vi "ScanAction.vi"(8 "error in (no error)":errorcluster caption="entrée d'erreur (pas d'erreur)", 9 "IndicePoint":i32, 11 "Dev In":refnum<class "KlingerMotor.lvclass"> caption="DNL_LabVIEW Object in") -> (0 "error out":errorcluster caption="sortie d'erreur", 2 "ScanParsOut":dbl[](array[numeric]), 3 "Dev Out":refnum<class "KlingerMotor.lvclass"> caption="DNL_LabVIEW Object out")   [LabVIEW 2012, in "KlingerMotor.lvclass"]
uses:
  KlingerMotor.lvclass
  KlingerMotor.lvclass/KlingerMotor.ctl
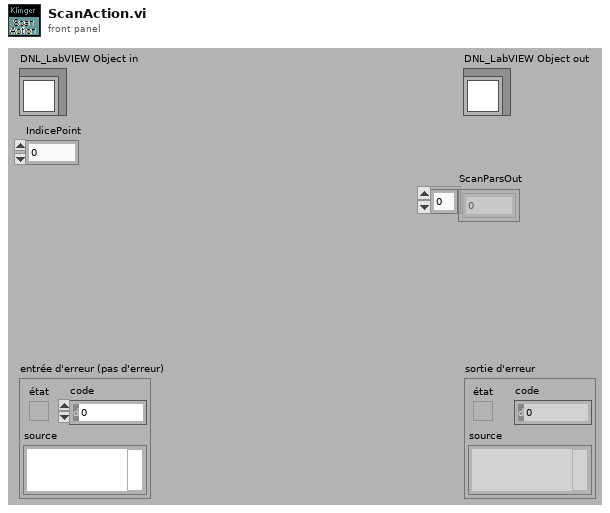
[diagram p1: front panel]
types:
  T1 = cluster{"Position Ref":refnum<vi>, "Moving Ref":refnum<vi>, "PLimRef":refnum<vi>, "NLimRef":refnum<vi>}
  T2 = typedef "KlingerMotor.lvclass/KlingerMotor_Func.ctl" = enum16{"Positions (mm)", "Position (ps)", "ReadWPos (ps)", "ReadWPos (mm)", "ReadZPos (ps)", "ReadZPos (mm)"}
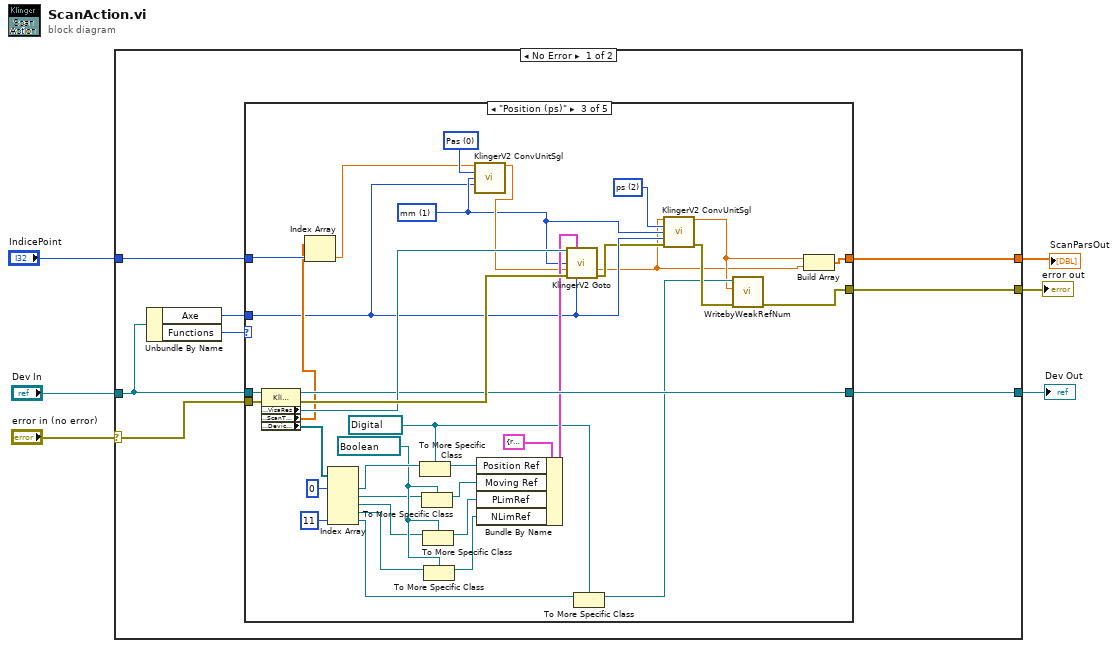
[diagram p0: block diagram]
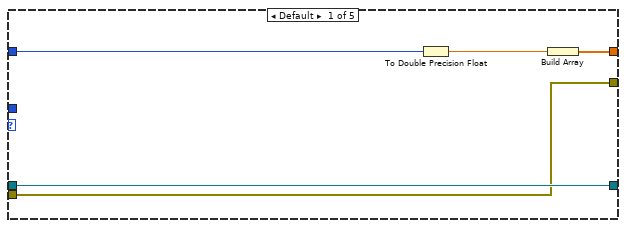
[diagram p2: hidden frame]
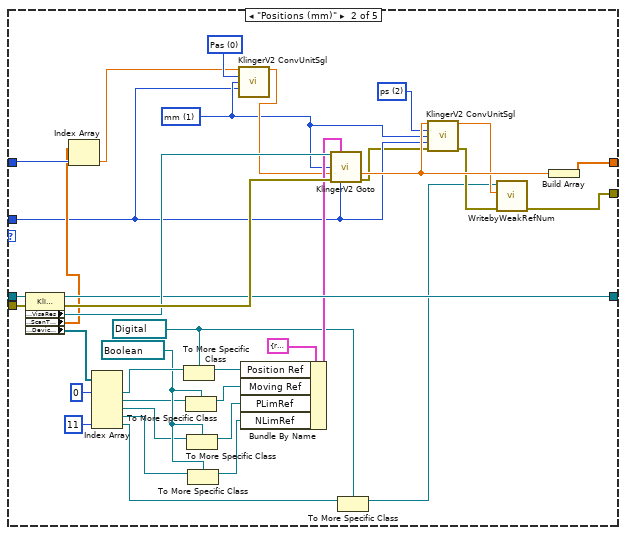
[diagram p3: hidden frame]
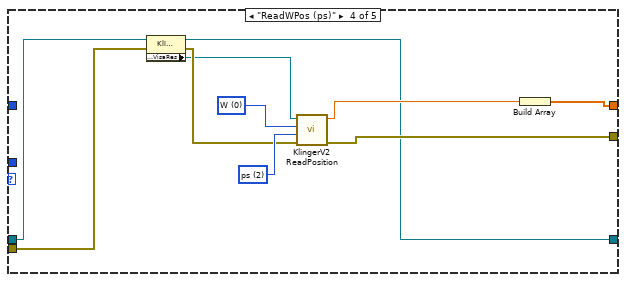
[diagram p4: hidden frame]
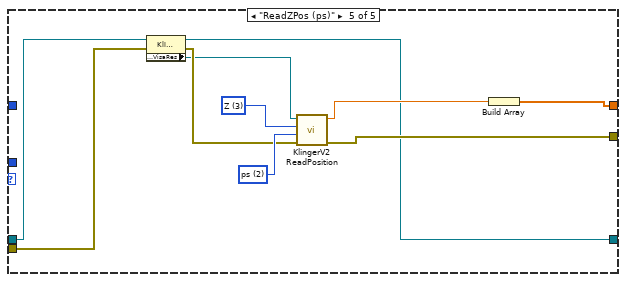
[diagram p5: hidden frame]
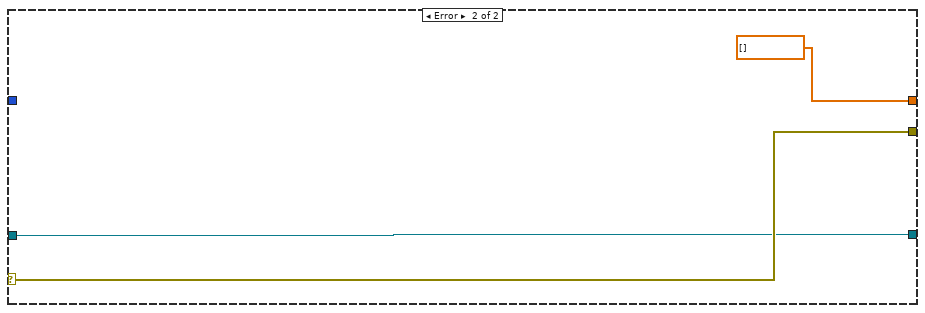
[diagram p6: hidden frame]
diagram:
  n1 = case shown="No Error" "error in (no error)" {
    selector: "error in (no error)" -> [w11 w114]
    tunnel: "Dev In" -> [w12 w113]
    tunnel: [w10 dbl[] []] -> w1
    tunnel: [w9 w114] -> w4
    tunnel: [w8 w113] -> w3
    tunnel: "IndicePoint" -> [w13 _]
    frame No Error {
      n2 = Unbundle By Name(w12) -> ("Axe"=w7:u8, "Functions"=w14:T2)
      n3 = case shown="\"Position (ps)\"" w14 {
        tunnel: [w15 w20 w57 w92 w102] -> w10
        tunnel: w13 -> [w19 w51 w87 _ _]
        tunnel: [w17 w50 w86 w93 w103] -> w8
        tunnel: w12 -> [w17 w55 w91 w96 w106]
        tunnel: w11 -> [w16 w54 w90 w97 w107]
        tunnel: [w16 w25 w62 w94 w104] -> w9
        tunnel: w7 -> [_ w29 w66 _ _]
        frame Default {
          n4 = To Double Precision Float(number=w19) -> (double precision float=w18:dbl)
          n5 = Build Array(w18) -> (w15:dbl[])
        }
        frame "Positions (mm)" {
          w31 = u8 2 items=["Pas", "mm", "ps", "Degré (°)"] ("UnitDem")
          w35 = u8 0 items=["Pas", "mm", "ps", "Degré (°)"] ("UnitDem")
          w42 = refnum<vi> refnum ("Moving Ref")
          w22 = refnum<vi> refnum ("Position Ref")
          w30 = u8 1 items=["Pas", "mm", "ps"] ("UnitDem")
          n6 = property class="KlingerMotor.lvclass"(reference=w55, error in=w54) -> (reference out=w50:refnum<class "KlingerMotor.lvclass">, error out=w53:errorcluster, "Accessor:VisaRes"=w52:refnum<visa-resource-name>, "Accessor:ScanTable"=w49:dbl[], "Accessor:DeviceCtrl"=w46:refnum<vi>[])
          n7 = Index Array(array=w49, index=w51) -> (element=w34:dbl)
          n8 = Index Array(array=w46, index #1=0 ("index"), index #5=11 ("index")) -> (element #1=w45:refnum<vi>, element #2=w41:refnum<vi>, element #3=w40:refnum<vi>, element #4=w39:refnum<vi>, element #5=w23:refnum<vi>)  [unwired: 3 in]
          n9 = To More Specific Class(target class=w22, reference=w45) -> (specific class reference=w43:refnum<vi>)  [unwired: 1 in, 1 out]
          n10 = To More Specific Class(target class=w42, reference=w41) -> (specific class reference=w38:refnum<vi>)  [unwired: 1 in, 1 out]
          n11 = To More Specific Class(target class=w42, reference=w40) -> (specific class reference=w37:refnum<vi>)  [unwired: 1 in, 1 out]
          n12 = To More Specific Class(target class=w42, reference=w39) -> (specific class reference=w36:refnum<vi>)  [unwired: 1 in, 1 out]
          n13 = call <userlib>:"KlingerV2 ConvUnitSgl.vi"("ParamAct"=w34, "UnitDem"=w35, "UnitAct"=w30, "Axe"=w29) -> ("ParamDem"=w33:dbl)  [unwired: 10 in, 1 out]
          n14 = Bundle By Name(cluster=T1 {"Position Ref"=refnum, "Moving Ref"=refnum, "PLimRef"=refnum, "NLimRef"=refnum} ("Ctrl Refs"), "Position Ref"=w43, "Moving Ref"=w38, "PLimRef"=w37, "NLimRef"=w36) -> (w47:T1)
          n15 = call <userlib>:"KlingerV2 Goto.vi"("VISA Rsrc"=w52, "Ctrl Refs"=w47, "UnitDem"=w30, "PosDem"=w33, "error in"=w53, "Axe"=w29) -> ("Position Out"=w32:dbl, "error out"=w28:errorcluster)  [unwired: 3 in, 5 out]
          n16 = To More Specific Class(target class=w22, reference=w23) -> (specific class reference=w21:refnum<vi>)  [unwired: 1 in, 1 out]
          n17 = call <userlib>:"KlingerV2 ConvUnitSgl.vi"("ParamAct"=w32, "UnitDem"=w31, "UnitAct"=w30, "Axe"=w29, "error in"=w28) -> ("ParamDem"=w24:dbl, "error out"=w26:errorcluster)  [unwired: 9 in]
          n18 = call <userlib>:"WritebyWeakRefNum.vi"("error in"=w26, "Valeur"=w24, "Control Ref"=w21) -> ("error out"=w25:errorcluster)  [unwired: 8 in]
          n19 = Build Array(w32) -> (w20:dbl[])
        }
        frame "Position (ps)" {
          w68 = u8 2 items=["Pas", "mm", "ps", "Degré (°)"] ("UnitDem")
          w71 = u8 0 items=["Pas", "mm", "ps", "Degré (°)"] ("UnitDem")
          w78 = refnum<vi> refnum ("Moving Ref")
          w60 = refnum<vi> refnum ("Position Ref")
          w67 = u8 1 items=["Pas", "mm", "ps"] ("UnitDem")
          n20 = property class="KlingerMotor.lvclass"(reference=w91, error in=w90) -> (reference out=w86:refnum<class "KlingerMotor.lvclass">, error out=w89:errorcluster, "Accessor:VisaRes"=w88:refnum<visa-resource-name>, "Accessor:ScanTable"=w85:dbl[], "Accessor:DeviceCtrl"=w82:refnum<vi>[])
          n21 = Index Array(array=w85, index=w87) -> (element=w70:dbl)
          n22 = Index Array(array=w82, index #1=0 ("index"), index #5=11 ("index")) -> (element #1=w81:refnum<vi>, element #2=w77:refnum<vi>, element #3=w76:refnum<vi>, element #4=w75:refnum<vi>, element #5=w61:refnum<vi>)  [unwired: 3 in]
          n23 = To More Specific Class(target class=w60, reference=w81) -> (specific class reference=w79:refnum<vi>)  [unwired: 1 in, 1 out]
          n24 = To More Specific Class(target class=w78, reference=w77) -> (specific class reference=w74:refnum<vi>)  [unwired: 1 in, 1 out]
          n25 = To More Specific Class(target class=w78, reference=w76) -> (specific class reference=w73:refnum<vi>)  [unwired: 1 in, 1 out]
          n26 = To More Specific Class(target class=w78, reference=w75) -> (specific class reference=w72:refnum<vi>)  [unwired: 1 in, 1 out]
          n27 = call <userlib>:"KlingerV2 ConvUnitSgl.vi"("ParamAct"=w70, "UnitDem"=w71, "UnitAct"=w67, "Axe"=w66) -> ("ParamDem"=w69:dbl)  [unwired: 10 in, 1 out]
          n28 = Bundle By Name(cluster=T1 {"Position Ref"=refnum, "Moving Ref"=refnum, "PLimRef"=refnum, "NLimRef"=refnum} ("Ctrl Refs"), "Position Ref"=w79, "Moving Ref"=w74, "PLimRef"=w73, "NLimRef"=w72) -> (w83:T1)
          n29 = call <userlib>:"KlingerV2 Goto.vi"("VISA Rsrc"=w88, "Ctrl Refs"=w83, "UnitDem"=w67, "PosDem"=w69, "error in"=w89, "Axe"=w66) -> ("Position Out"=w56:dbl, "error out"=w65:errorcluster)  [unwired: 3 in, 5 out]
          n30 = To More Specific Class(target class=w60, reference=w61) -> (specific class reference=w59:refnum<vi>)  [unwired: 1 in, 1 out]
          n31 = call <userlib>:"KlingerV2 ConvUnitSgl.vi"("ParamAct"=w56, "UnitDem"=w68, "UnitAct"=w67, "Axe"=w66, "error in"=w65) -> ("ParamDem"=w58:dbl, "error out"=w63:errorcluster)  [unwired: 9 in]
          n32 = call <userlib>:"WritebyWeakRefNum.vi"("error in"=w63, "Valeur"=w58, "Control Ref"=w59) -> ("error out"=w62:errorcluster)  [unwired: 8 in]
          n33 = Build Array(w58, w56) -> (w57:dbl[])
        }
        frame "ReadWPos (ps)" {
          w101 = u8 0 items=["W", "X", "Y", "Z"] ("Axe")
          w100 = u8 2 items=["Pas", "mm", "ps", "Degré (°)"] ("UnitDem")
          n34 = property class="KlingerMotor.lvclass"(reference=w96, error in=w97) -> (reference out=w93:refnum<class "KlingerMotor.lvclass">, error out=w99:errorcluster, "Accessor:VisaRes"=w98:refnum<visa-resource-name>)
          n35 = call <userlib>:"KlingerV2 ReadPosition.vi"("error in"=w99, "UnitDem"=w100, "Axe"=w101, "VISA Rsrc"=w98) -> ("error out"=w94:errorcluster, "Position"=w95:dbl)  [unwired: 1 in, 5 out]
          n36 = Build Array(w95) -> (w92:dbl[])
        }
        frame "ReadZPos (ps)" {
          w111 = u8 3 items=["W", "X", "Y", "Z"] ("Axe")
          w110 = u8 2 items=["Pas", "mm", "ps", "Degré (°)"] ("UnitDem")
          n37 = property class="KlingerMotor.lvclass"(reference=w106, error in=w107) -> (reference out=w103:refnum<class "KlingerMotor.lvclass">, error out=w109:errorcluster, "Accessor:VisaRes"=w108:refnum<visa-resource-name>)
          n38 = call <userlib>:"KlingerV2 ReadPosition.vi"("error in"=w109, "UnitDem"=w110, "Axe"=w111, "VISA Rsrc"=w108) -> ("error out"=w104:errorcluster, "Position"=w105:dbl)  [unwired: 1 in, 5 out]
          n39 = Build Array(w105) -> (w102:dbl[])
        }
      }
    }
    frame Error {
    }
  }
  "error out" <- w4
  "Dev Out" <- w3
  "ScanParsOut" <- w1
